vi "Qudi_MulticolourScanTask.vi"(3 "N Z positions":i32) -> ()   [LabVIEW 2015]
uses:
  <vilib>/rvi/Emulation/niFpgaGetClockAttributes.vi
  <vilib>/rvi/Emulation/niFpgaSctlEmulationGetInTimedLoop.vi
  <vilib>/rvi/Emulation/niFpgaEmulationReportErrorSimple.vi
  <vilib>/rvi/eio/common/nirviEmuTemplateMethod_errors.vi
  <vilib>/rvi/Emulation/niFpgaProcessEmulError.vi
  <vilib>/rvi/Emulation/niFpgaCriticalErrorInLSC.vi
  <vilib>/eio/EIONode/EIONode.xnode
panel:
  in  "exposure_time_ms":u16
  in  "stop":bool
  out "n cycles":i32
  out "Images acquired":i32
  in  "Laser lines":i8[](array[numeric])=[0, 0, 0, 0, 0]
  in  "N laser lines":i32
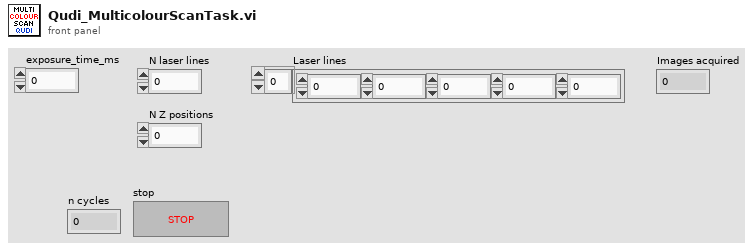
[diagram p1: front panel]
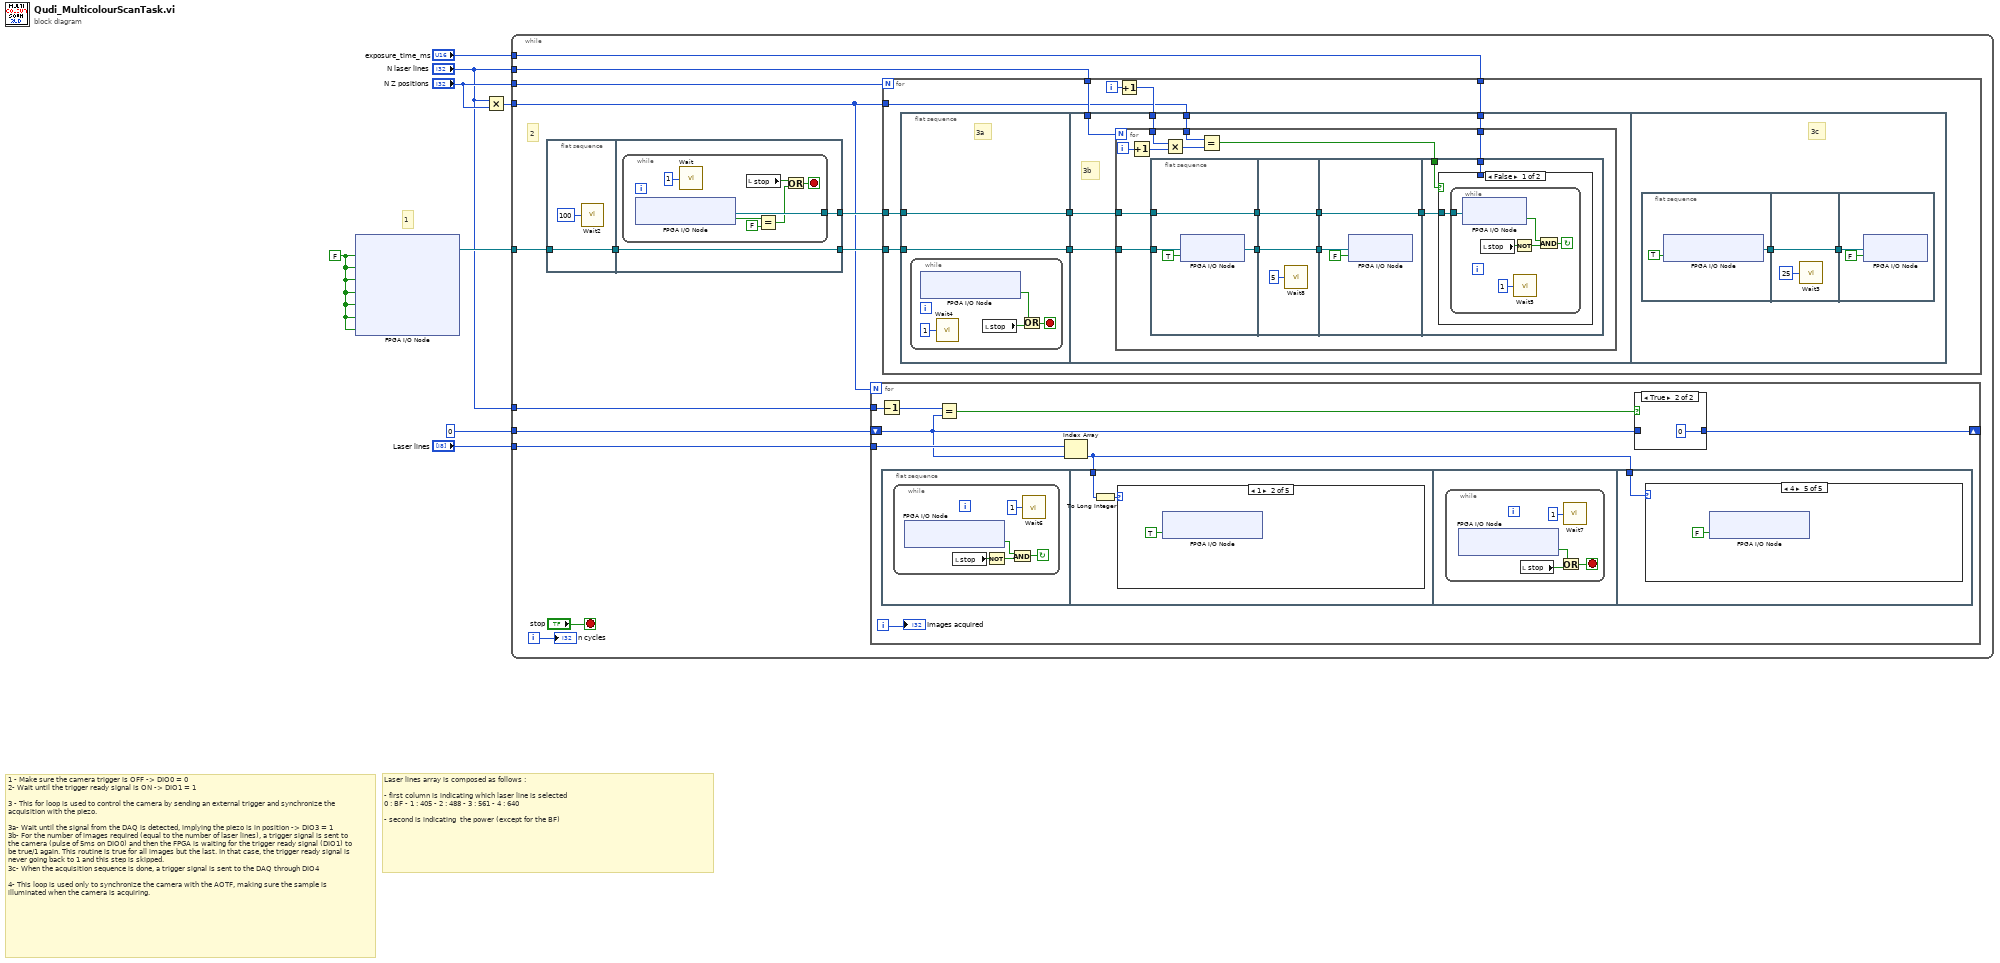
[diagram p0: block diagram]
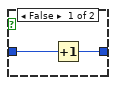
[diagram p2: hidden frame]
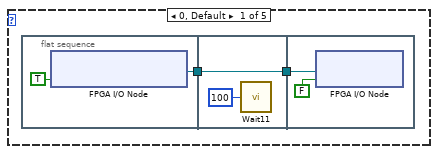
[diagram p3: hidden frame]
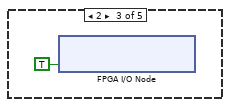
[diagram p4: hidden frame]
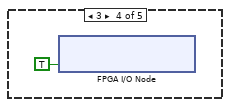
[diagram p5: hidden frame]
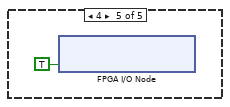
[diagram p6: hidden frame]
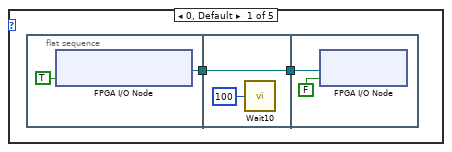
[diagram p7: hidden frame]
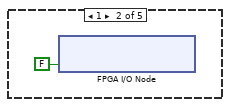
[diagram p8: hidden frame]
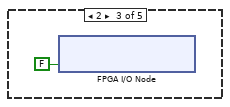
[diagram p9: hidden frame]
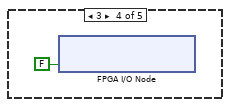
[diagram p10: hidden frame]
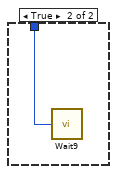
[diagram p11: hidden frame]
diagram:
  w1 = FALSE ("Connector0/DIO0")
  # "Laser lines array is composed as follows :\n\n- first column is indicating which laser line is selected \n0 : BF - 1 : 405 - 2 : 488 - 3 : 561 - 4 : 640\n\n- second is indicating  the power (except for the BF)"
  # "1"
  # "1 - Make sure the camera trigger is OFF -> DIO0 = 0\n2- Wait until the trigger ready signal is ON -> DIO1 = 1\n\n3 - This for loop is used to control the camera by sending an external trigger and synchronize the acquisition with the piezo.\n\n3a- Wait until the signal from the DAQ is detected, implying the piezo is in position -> DIO3 = 1 \n3b- For the number of images required (equal to the number of laser lines), a trigger signal is sent to the camera (pulse of 5ms on DIO0) and then the FPGA is waiting for the trigger ready signal (DIO1) to be true/1 again. This routine is true for all images but the last. In that case, the trigger ready signal is never going back to 1 and this step is skipped. \n3c- When the acquisition sequence is done, a trigger signal is sent to the DAQ through DIO4\n\n4- This loop is used only to synchronize the camera with the AOTF, making sure the sample is illuminated when the camera is acquiring."
  n1 = xnode "FPGA I/O Node"("Connector0/DIO0"=w1, "Connector0/DIO6"=w1, "Connector0/DIO7"=w1, "Connector0/DIO8"=w1, "Connector0/DIO9"=w1, "Connector0/DIO10"=w1, "Connector0/DIO5"=w1) -> ("FPGA I/O Out"=w8:refnum<k21>)  [unwired: 7 in, 6 out]
  n2 = Multiply(x="N laser lines", y="N Z positions") -> (x*y=w4:i32)
  n3 = while {
    tunnel: w8 -> [w20]
    tunnel: "Laser lines" -> [w17]
    tunnel: 0 -> [w16]
    tunnel: "N Z positions" -> [w15]
    tunnel: "N laser lines" -> [w13]
    tunnel: w4 -> [w12]
    tunnel: "N laser lines" -> [w11]
    tunnel: "exposure_time_ms" -> [w10]
    i -> [w14]
    stop <- "stop" stop-if-true
    # "2"
    n4 = flat-sequence {
      tunnel: w20 -> [w70]
      tunnel: [w70] -> w21
      tunnel: w21 -> [w72]
      tunnel: [w72] -> w19
      tunnel: [w71] -> w18
      frame #0 {
        n5 = call "Wait2"("Count(uSec)"=u8 100 ("Count(mSec)")) -> ()  [unwired: 1 out]
      }
      frame #1 {
        n6 = while {
          tunnel: [w79] -> w71
          stop <- w74 stop-if-true
          n7 = xnode "FPGA I/O Node"() -> ("Connector0/DIO1"=w78:bool, "FPGA I/O Out"=w79:refnum<k21>)  [unwired: 1 in]
          n8 = call "Wait"("Count(mSec)"=u8 1) -> ()  [unwired: 1 out]
          n9 = local read "stop"() -> (w75:bool)
          n10 = Equal?(x=w78, y=FALSE) -> (x = y?=w76:bool)
          n11 = Or(x=w75, y=w76) -> (x .or. y?=w74:bool)
        }
      }
    }
    n12 = for {
      N: w12 -> [_]
      shift-right: [w27] -> _
      shift-left: w16 -> [w25]
      tunnel: w17 -> [w26]
      tunnel: w11 -> [w24]
      i -> [w22]
      n13 = Decrement(x=w24) -> (x-1=w23:i32)
      n14 = flat-sequence {
        tunnel: w29 -> [w38]
        tunnel: w29 -> [w56]
        frame #0 {
          n15 = while {
            stop <- w34 continue-if-true
            n16 = xnode "FPGA I/O Node"() -> ("Connector0/DIO2"=w35:bool)  [unwired: 1 in, 1 out]
            n17 = local read "stop"() -> (w36:bool)
            n18 = Not(x=w36) -> (.not. x?=w37:bool)
            n19 = And(x=w35, y=w37) -> (x .and. y?=w34:bool)
            n20 = call "Wait6"("Count(mSec)"=u8 1) -> ()  [unwired: 1 out]
          }
        }
        frame #1 {
          n21 = To Long Integer(number=w38) -> (32bit integer=w39:i32)
          n22 = case shown="1" w39 {
            frame 0, Default {
              n23 = flat-sequence {
                tunnel: [w42] -> w41
                tunnel: w41 -> [w44]
                tunnel: [w44] -> w40
                tunnel: w40 -> [w47]
                frame #0 {
                  n24 = xnode "FPGA I/O Node"("Connector0/DIO5"=TRUE) -> ("FPGA I/O Out"=w42:refnum<k21>)  [unwired: 1 in]
                }
                frame #1 {
                  n25 = call "Wait11"("Count(uSec)"=u32 100) -> ()  [unwired: 1 out]
                }
                frame #2 {
                  n26 = xnode "FPGA I/O Node"("I/O Item"=FALSE, "FPGA I/O In"=w47) -> ()  [unwired: 1 out]
                }
              }
            }
            frame 1 {
              n27 = xnode "FPGA I/O Node"("Connector0/DIO6"=TRUE) -> ()  [unwired: 1 in, 1 out]
            }
            frame 2 {
              n28 = xnode "FPGA I/O Node"("Connector0/DIO6"=TRUE) -> ()  [unwired: 1 in, 1 out]
            }
            frame 3 {
              n29 = xnode "FPGA I/O Node"("Connector0/DIO8"=TRUE) -> ()  [unwired: 1 in, 1 out]
            }
            frame 4 {
              n30 = xnode "FPGA I/O Node"("Connector0/DIO9"=TRUE ("Connector0/DIO6")) -> ()  [unwired: 1 in, 1 out]
            }
          }
        }
        frame #2 {
          n31 = while {
            stop <- w53 stop-if-true
            n32 = xnode "FPGA I/O Node"() -> ("Connector0/DIO2"=w54:bool)  [unwired: 1 in, 1 out]
            n33 = local read "stop"() -> (w55:bool)
            n34 = Or(x=w54, y=w55) -> (x .or. y?=w53:bool)
            n35 = call "Wait7"("Count(mSec)"=u8 1) -> ()  [unwired: 1 out]
          }
        }
        frame #3 {
          n36 = case shown="4" w56 {
            frame 0, Default {
              n37 = flat-sequence {
                tunnel: [w59] -> w58
                tunnel: w58 -> [w61]
                tunnel: [w61] -> w57
                tunnel: w57 -> [w64]
                frame #0 {
                  n38 = xnode "FPGA I/O Node"("Connector0/DIO5"=TRUE) -> ("FPGA I/O Out"=w59:refnum<k21>)  [unwired: 1 in]
                }
                frame #1 {
                  n39 = call "Wait10"("Count(uSec)"=u32 100) -> ()  [unwired: 1 out]
                }
                frame #2 {
                  n40 = xnode "FPGA I/O Node"("I/O Item"=FALSE, "FPGA I/O In"=w64) -> ()  [unwired: 1 out]
                }
              }
            }
            frame 1 {
              n41 = xnode "FPGA I/O Node"("Connector0/DIO6"=FALSE) -> ()  [unwired: 1 in, 1 out]
            }
            frame 2 {
              n42 = xnode "FPGA I/O Node"("Connector0/DIO7"=FALSE) -> ()  [unwired: 1 in, 1 out]
            }
            frame 3 {
              n43 = xnode "FPGA I/O Node"("Connector0/DIO8"=FALSE) -> ()  [unwired: 1 in, 1 out]
            }
            frame 4 {
              n44 = xnode "FPGA I/O Node"("Connector0/DIO9"=FALSE) -> ()  [unwired: 1 in, 1 out]
            }
          }
        }
      }
      n45 = Equal?(x=w23, y=w25) -> (x = y?=w28:bool)
      n46 = Index Array(array=w26, index=w25) -> (element=w29:i8)
      n47 = case shown="True" w28 {
        tunnel: w25 -> [w31 _]
        tunnel: [w30 0] -> w27
        frame False {
          n48 = Increment(x=w31) -> (x+1=w30:i32)
        }
        frame True {
        }
      }
      "Images acquired" <- w22
    }
    n49 = for {
      N: w15 -> [_]
      tunnel: w19 -> [w87]
      tunnel: w18 -> [w88]
      tunnel: w13 -> [w83]
      tunnel: w12 -> [w81]
      tunnel: w10 -> [w80]
      i -> [w84]
      n50 = flat-sequence {
        tunnel: w87 -> [w89]
        tunnel: w88 -> [w90]
        tunnel: [w90] -> w86
        tunnel: [w89] -> w85
        tunnel: w86 -> [w100]
        tunnel: w85 -> [w99]
        tunnel: w83 -> [w98]
        tunnel: w82 -> [w97]
        tunnel: w81 -> [w96]
        tunnel: w80 -> [w95]
        frame #0 {
          # "3a"
          n51 = while {
            stop <- w92 stop-if-true
            n52 = xnode "FPGA I/O Node"() -> ("Connector0/DIO3"=w93:bool)  [unwired: 1 in, 1 out]
            n53 = call "Wait4"("Count(mSec)"=u8 1) -> ()  [unwired: 1 out]
            n54 = local read "stop"() -> (w94:bool)
            n55 = Or(x=w93, y=w94) -> (x .or. y?=w92:bool)
          }
        }
        frame #1 {
          # "3b"
          n56 = for {
            N: w98 -> [_]
            tunnel: w100 -> [w109]
            tunnel: w99 -> [w108]
            tunnel: w97 -> [w105]
            tunnel: w96 -> [w103]
            tunnel: w95 -> [w101]
            i -> [w107]
            n57 = Increment(x=w107) -> (x+1=w106:i32)
            n58 = flat-sequence {
              tunnel: [w117] -> w114
              tunnel: [w115] -> w113
              tunnel: w108 -> [w116]
              tunnel: w109 -> [w115]
              tunnel: w114 -> [w121]
              tunnel: [w121] -> w112
              tunnel: [w120] -> w111
              tunnel: w113 -> [w120]
              tunnel: w112 -> [w123]
              tunnel: [w122] -> w110
              tunnel: w111 -> [w122]
              tunnel: w110 -> [w127]
              tunnel: w102 -> [w126]
              tunnel: w101 -> [w125]
              frame #0 {
                n59 = xnode "FPGA I/O Node"("I/O Item"=TRUE ("Connector0/DIO0"), "FPGA I/O In"=w116) -> ("FPGA I/O Out"=w117:refnum<k21>)
              }
              frame #1 {
                n60 = call "Wait8"("Count(mSec)"=u8 5) -> ()  [unwired: 1 out]
              }
              frame #2 {
                n61 = xnode "FPGA I/O Node"("I/O Item"=FALSE ("Connector0/DIO0"), "FPGA I/O In"=w123) -> ()  [unwired: 1 out]
              }
              frame #3 {
                n62 = case shown="False" w126 {
                  tunnel: w127 -> [w128 _]
                  tunnel: w125 -> [_ w135]
                  frame False {
                    n63 = while {
                      tunnel: w128 -> [w134]
                      stop <- w130 continue-if-true
                      n64 = xnode "FPGA I/O Node"("FPGA I/O In"=w134) -> ("I/O Item"=w131:bool)  [unwired: 1 out]
                      n65 = local read "stop"() -> (w133:bool)
                      n66 = Not(x=w133) -> (.not. x?=w132:bool)
                      n67 = call "Wait5"("Count(mSec)"=u8 1) -> ()  [unwired: 1 out]
                      n68 = And(x=w131, y=w132) -> (x .and. y?=w130:bool)
                    }
                  }
                  frame True {
                    n69 = call "Wait9"("Count(mSec)"=w135) -> ()  [unwired: 1 out]
                  }
                }
              }
            }
            n70 = Multiply(x=w105, y=w106) -> (x*y=w104:i32)
            n71 = Equal?(x=w103, y=w104) -> (x = y?=w102:bool)
          }
        }
        frame #2 {
          # "3c"
          n72 = flat-sequence {
            tunnel: [w139] -> w137
            tunnel: w137 -> [w140]
            tunnel: [w140] -> w136
            tunnel: w136 -> [w142]
            frame #0 {
              n73 = xnode "FPGA I/O Node"("Connector0/DIO4"=TRUE) -> ("FPGA I/O Out"=w139:refnum<k21>)  [unwired: 1 in]
            }
            frame #1 {
              n74 = call "Wait3"("Count(mSec)"=u8 25) -> ()  [unwired: 1 out]
            }
            frame #2 {
              n75 = xnode "FPGA I/O Node"("I/O Item"=FALSE ("Connector0/DIO0"), "FPGA I/O In"=w142) -> ()  [unwired: 1 out]
            }
          }
        }
      }
      n76 = Increment(x=w84) -> (x+1=w82:i32)
    }
    "n cycles" <- w14
  }
